vi "DeConAPD1FGV.vi"(8 "Error In":errorcluster, 10 "Operation (Read)":enum16{"Read", "Write"}(ring), 11 "APDClass in":T1) -> (0 "Error Out":errorcluster, 3 "APDClass out":T1)   [LabVIEW 2019]
uses:
  DotNetDecon/APD.ctl
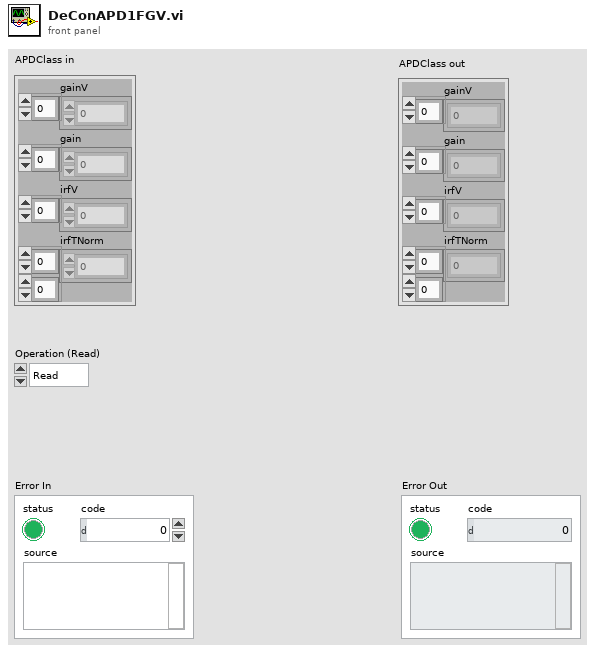
[diagram p1: front panel]
types:
  T1 = typedef "APD.ctl" = cluster{"gainV":dbl[], "gain":dbl[], "irfV":dbl[], "irfTNorm":dbl[][]}
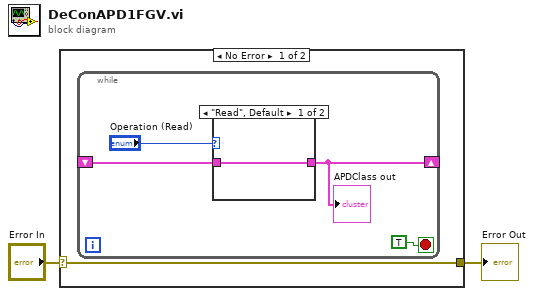
[diagram p0: block diagram]
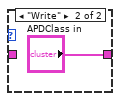
[diagram p2: hidden frame]
diagram:
  n1 = case shown="No Error" "Error In" {
    selector: "Error In" -> [w3 w10]
    tunnel: [w3 w10] -> w1
    frame No Error {
      n2 = while {
        shift-right: [w5] -> _
        shift-left: _ -> [w4]
        stop <- TRUE stop-if-true
        n3 = case shown="\"Read\", Default" "Operation (Read)" {
          tunnel: [w8 "APDClass in"] -> w5
          tunnel: w4 -> [w8 _]
          frame "Read", Default {
          }
          frame "Write" {
          }
        }
        "APDClass out" <- w5
      }
    }
    frame Error {
    }
  }
  "Error Out" <- w1
